vi "Deserialize an Object.vi"() -> ()   [LabVIEW 2017]
doc: "Demonstrates the JSONtext Object Serializer by deserializing a LabVIEW Object from JSON."
uses:
  Generic Object Serializer/Generic Object Serializer.lvclass
  C:/Program Files (x86)/National Instruments/LabVIEW 2017/vi.lib/JDP Science/JSONtext/LVClass Serializer/JSONtext LVClass Serializer.lvclass
  Account/Account.lvclass
  c1b321db-ba44-4e46-b14b-83a8d0196014.vi
  <vilib>/JDP Science/JSONtext/JSON text to Variant.vi
panel:
  out "Summary":string
  out "error out":errorcluster
  in  "<JSON>":string="{\n  \"Email\":\"john.doe@example.com\",\n  \"Active\":true,\n  \"CreatedDate\":\"2021-04-03T06:30:00.000Z\",\n  \"Roles\":[\"User\",\"Admin\"]\n}"
  # "Overview\nDemonstrates the JSONtext Object Serializer by deserializing a LabVIEW Object from JSON.\n\nInstructions\nRun the VI"
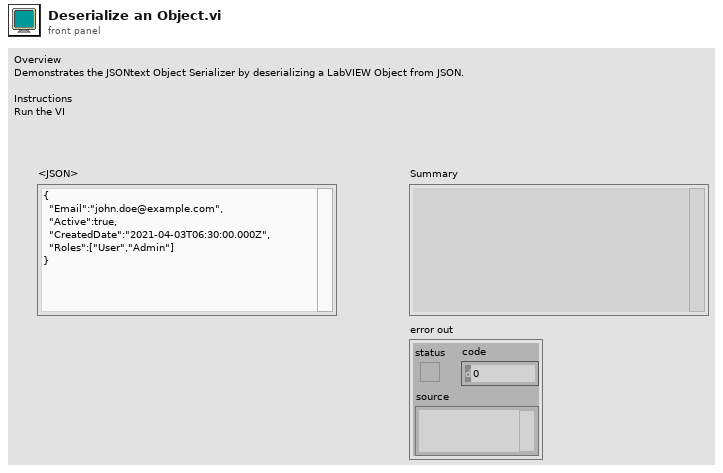
[diagram p1: front panel]
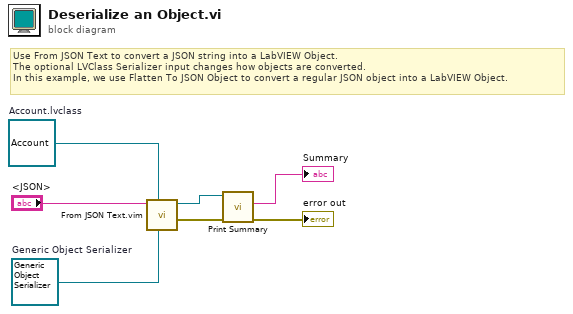
[diagram p0: block diagram]
diagram:
  w4 = refnum<class "Account.lvclass"> refnum  # Account.lvclass
  w6 = refnum<class "Generic Object Serializer.lvclass"> refnum  # Generic Object Serializer
  # "Use From JSON Text to convert a JSON string into a LabVIEW Object.\nThe optional LVClass Serializer input changes how objects are converted.\nIn this example, we use Flatten To JSON Object to convert a regular JSON object into a LabVIEW Object."
  n1 = call "From JSON Text.vim"("LVClass Serializer"=w6, "Data Type and Default Value"=w4, "JSON"="<JSON>") -> ("error out"=w7:errorcluster, "Data out"=w2:refnum<class "Account.lvclass">)  [unwired: 7 in]
  n2 = call "Print Summary.vi"("error in (no error)"=w7, "Account in"=w2) -> ("error out"=→"error out":errorcluster, "Summary"=→"Summary":string)  [unwired: 7 in, 1 out]
